vi "Init.vi"(8 "error in (no error)":errorcluster, 11 "Data in":refnum<class "Bus_Access.lvclass">) -> (0 "error out":errorcluster, 3 "Data out":refnum<class "Bus_Access.lvclass">)   [LabVIEW 2021, in "Bus_Access.lvclass"]
doc: "Abstract Data Classes 2.1.1.12\nTim Streeter - TSA\nCopyright (c) 2024, TSA"
uses:
  Bus_Access.lvclass
  Bus_Access.lvclass/Bus_Access.ctl
  Properties/Read Tag Root.vi
  Properties/Read Tags.vi
  Properties/Write Tags.vi
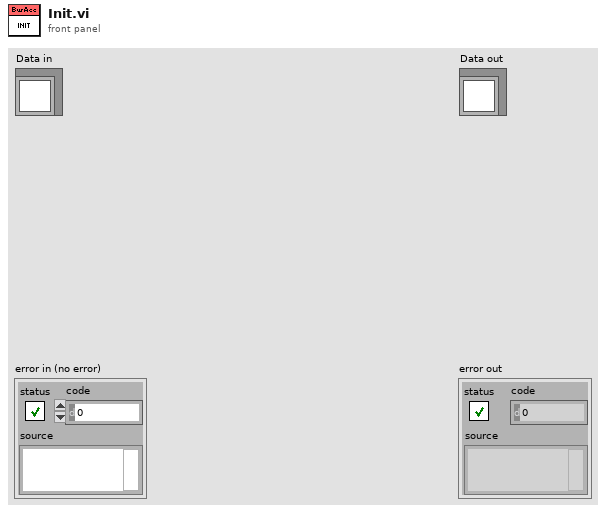
[diagram p1: front panel]
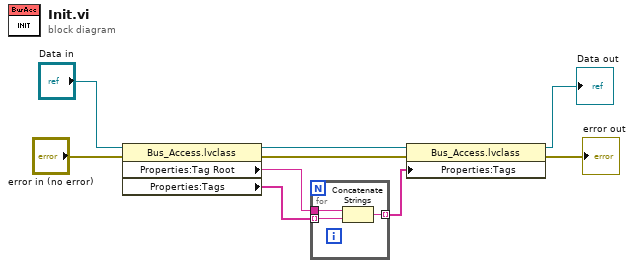
[diagram p0: block diagram]
diagram:
  n1 = property class="Bus_Access.lvclass"(reference="Data in", error in="error in (no error)") -> (reference out=w4:refnum<class "Bus_Access.lvclass">, error out=w5:errorcluster, "Properties:Tag Root"=w7:string, "Properties:Tags"=w6:string[])
  n2 = for {
    tunnel: w7 -> [w12]
    tunnel: w6 -> [w11] mode=indexing
    tunnel: [w10] -> w3 mode=indexing
    n3 = Concatenate Strings(w12, w11) -> (w10:string)
  }
  n4 = property class="Bus_Access.lvclass"(reference=w4, error in=w5, "Properties:Tags"=w3) -> (reference out=→"Data out":refnum<class "Bus_Access.lvclass">, error out=→"error out":errorcluster)
